vi "tcs shm issue Command exit Control LV.vi"(8 "error in (no error)":errorcluster, 11 "command_exitControl_Ctl":cluster{"state":u8}) -> (0 "error out":errorcluster, 2 "function return":i32, 3 "command_exitControl_Ctl out":cluster{"state":u8})   [LabVIEW 2016, in "SALLV_tcs.lvlib"]
doc: "int tcs_shm_issueCommand_exitControlLV(tcs_command_exitControlLV *command_exitControl_Ctl );"
uses:
  SALLV_tcs.lvlib
  SALLV_tcs.so
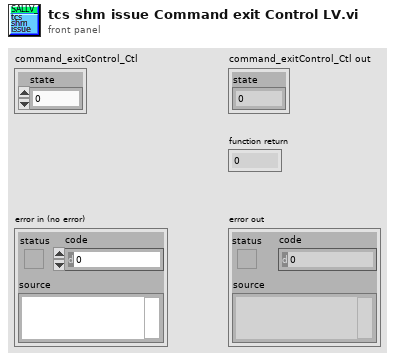
[diagram p1: front panel]
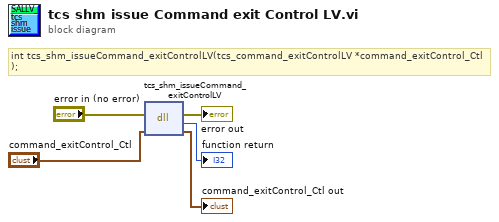
[diagram p0: block diagram]
diagram:
  # "int tcs_shm_issueCommand_exitControlLV(tcs_command_exitControlLV *command_exitControl_Ctl );"
  n1 = dll-call lib="home/plotz/SALLV_tcs/SALLV_tcs.*" fn="tcs_shm_issueCommand_exitControlLV"(error in="error in (no error)", "command_exitControl_Ctl"="command_exitControl_Ctl") -> (error out=→"error out":errorcluster, →"function return":i32, "command_exitControl_Ctl"=→"command_exitControl_Ctl out":cluster{"state":u8})  [unwired: 2 in, 1 out]
